vi "v5.51.vi"() -> ()   [LabVIEW 2018]
uses:
  <vilib>/DAQmx/read.llb/DAQmx Read (Analog 1D DBL NChan 1Samp).vi
  <extravilib>/ChannelInstances/Lossy Stream-c(a[.](c(dbl,dbl,dbl,dbl)),stamp,a[.](dbl),c(dbl,dbl,dbl,dbl,dbl,dbl,dbl))/Read With Abort.vi
  <extravilib>/ChannelInstances/High Speed Stream-c(a[.](c(dbl,dbl,dbl,dbl)),stamp,a[.](dbl),c(dbl,dbl,dbl,dbl,dbl,dbl,dbl))/_Read For Replicate.vi
  <extravilib>/ChannelInstances/Lossy Stream-c(a[.](c(dbl,dbl,dbl,dbl)),stamp,a[.](dbl),c(dbl,dbl,dbl,dbl,dbl,dbl,dbl))/Write With Abort.vi
  <extravilib>/ChannelInstances/Lossy Stream-c(a[.](c(dbl,dbl,dbl,dbl)),stamp,a[.](dbl),c(dbl,dbl,dbl,dbl,dbl,dbl,dbl))/EndpointRead.vi
  <extravilib>/ChannelInstances/Lossy Stream-c(a[.](c(dbl,dbl,dbl,dbl)),stamp,a[.](dbl),c(dbl,dbl,dbl,dbl,dbl,dbl,dbl))/Endpoint.vi
  <extravilib>/ChannelInstances/Lossy Stream-c(a[.](c(dbl,dbl,dbl,dbl)),stamp,a[.](dbl),c(dbl,dbl,dbl,dbl,dbl,dbl,dbl))/Instantiate.vi
  <extravilib>/ChannelInstances/Lossy Stream-c(a[.](c(dbl,dbl,dbl,dbl)),stamp,a[.](dbl),c(dbl,dbl,dbl,dbl,dbl,dbl,dbl))/)Channel.vi
  <resource>/ChannelSupport/_ChannelSupport/WaitIfNeeded.vi
  <extravilib>/ChannelInstances/High Speed Stream-c(a[.](c(dbl,dbl,dbl,dbl)),stamp,a[.](dbl),c(dbl,dbl,dbl,dbl,dbl,dbl,dbl))/Instantiate.vi
  <extravilib>/ChannelInstances/High Speed Stream-c(a[.](c(dbl,dbl,dbl,dbl)),stamp,a[.](dbl),c(dbl,dbl,dbl,dbl,dbl,dbl,dbl))/)Channel.vi
  <extravilib>/ChannelInstances/High Speed Stream-c(a[.](c(dbl,dbl,dbl,dbl)),stamp,a[.](dbl),c(dbl,dbl,dbl,dbl,dbl,dbl,dbl))/Abort Signal/Init Signal.vi
  <vilib>/Utility/file.llb/Write Delimited Spreadsheet (string).vi
  <vilib>/DAQmx/create/channels.llb/DAQmx Create Channel (AI-Temperature-Thermocouple).vi
  <vilib>/DAQmx/configure/timing.llb/DAQmx Timing (Sample Clock).vi
  <vilib>/DAQmx/miscellaneous.llb/DAQmx Fill In Error Info.vi
  <extravilib>/ChannelInstances/High Speed Stream-c(a[.](c(dbl,dbl,dbl,dbl)),stamp,a[.](dbl),c(dbl,dbl,dbl,dbl,dbl,dbl,dbl)).lvlib
  <resource>/objmgr/daqmx.rc
  <extravilib>/ChannelInstances/Lossy Stream-c(a[.](c(dbl,dbl,dbl,dbl)),stamp,a[.](dbl),c(dbl,dbl,dbl,dbl,dbl,dbl,dbl)).lvlib
panel:
  out "Thermal Power [kJ/s]":dbl
  out "Equivalence Ratio":dbl
  out "Total Air Flow Required for \nStoichiometric Combustion":dbl
  out "Mixture AFR":dbl
  out "Total Fuel Flow [g/s]":dbl
  out "Total Air Flow [g/s]":dbl
  in  "Rig Temperature Tab Box":enum32{"Rig Temps Live", "Alarm Thresholds"}(tab)
  out "Rig Temperatures":T1
  in  "Rig Alarm Thresholds":T1
  out "DAQ Current Time":timestamp format="%<%X>T"
  in  "UI Refresh Rate (Hz)":u32=1 min=1 max=500 step=1
  out "Line Pressures":T2(graph)
  in  "Boondoggle":dbl(slide) scale=0.0..10.0
  out "Line Temperatures":T2(graph)
  in  "Species List":string[][](table)=[["Custom", "9999999999", ""], ["Methanol", "6.47", "19.93"], ["Butanol", "11.2", "33.075"], ["Propane", "15.67", "46.35"], ["Methane", "13.19", "50.00"], ["Hydrogen", "34.3", "119.96"], ["Ammonia", "6.0466", "22.5"], ["Pentane", "15.32", "45.36"], ["Butane", "14.98", "45.75"], ["Hexane", "15.24", "44.75"], ["Ethanol", "9", "26.70"], ["Empty (Not Used)", "0", "0"]]
  in  "Lines Tab Control\n(Don't delete)":enum32{"Live Data", "AFR Info", "Setup Lines"}(tab)
  out "Flowrate Data":T3(array[cluster])
  out "AFR Display":T4(array[cluster])
  in  "Line Setup":T5(array[cluster])
  out "Actual Sample Rate":dbl
  out "Export Timestamp":timestamp format="%<%H:%M:%S>T"
  out "UI Timestamp":timestamp format="%<%X\n%x>T"
  in  "file path (dialog if empty)":path
  out "Export Loop Status":T6(ring)
  in  "Start Recording?":bool
  in  "Stop Recording?":bool
  out "Aquisition\nLoop Status":T7(ring)
  in  "OK Button":bool
  in  "DAQ Properties":cluster{"Sample Rate [Hz]":dbl}={"Sample Rate [Hz]"=1.0} {"Sample Rate [Hz]" min=1.0 max=500.0 step=1.0}
  # "Rig Temperatures [ °C]"
  # "Rig Alarm Thresholds [ °C]"
  # "Live \n Live Line Data"
  # "Air-to-Fuel Ratios for each Line"
  # "Line Setup"
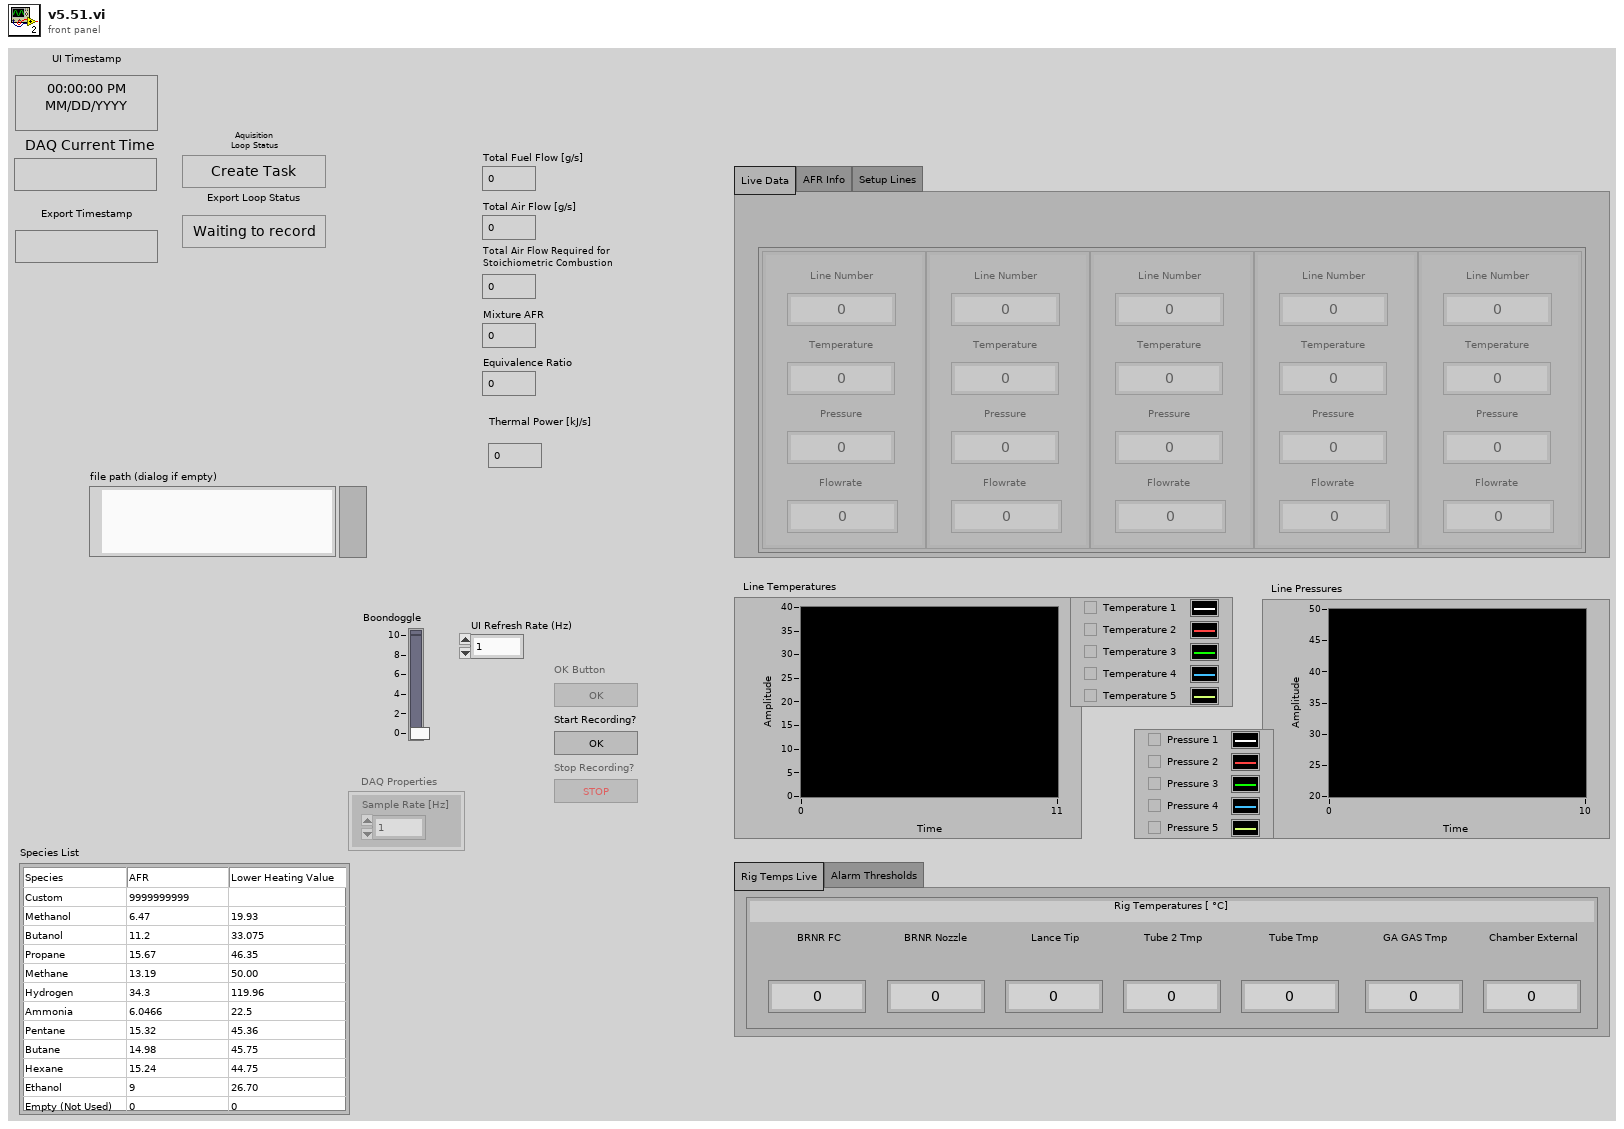
[diagram p1: front panel]
types:
  T1 = cluster{"BRNR FC":dbl, "BRNR Nozzle":dbl, "Lance Tip":dbl, "Tube 2 Tmp":dbl, "Tube Tmp":dbl, "GA GAS Tmp":dbl, "Chamber External":dbl}
  T2 = cluster{"[0]":dbl, "[1]":dbl, "[2]":dbl, "[3]":dbl, "[4]":dbl}
  T3 = cluster{"Line Number":dbl, "Temperature":dbl, "Pressure":dbl, "Flowrate":dbl}[]
  T4 = cluster{"Line Number":i32, "AFR":dbl, "Species":enum16{"Empty (Not used)", "Custom", "Air", "Methanol", "Ethanol", "Butanol", "Propane", "Methane", "Hydrogen", "Pentane", "Butane", "Hexane"}}[]
  T5 = cluster{"Custom AFR":dbl, "Species":enum16{"Empty (Not used)", "Custom", "Air", "Methanol", "Ethanol", "Butanol", "Propane", "Methane", "Hydrogen", "Pentane", "Butane", "Hexane"}, "Custom Lower Heating Value [kJ/kg]":dbl}[]
  T6 = enum16{"Waiting to record", "Creating Spreadsheet", "Recording", "Finished Recording"}
  T7 = enum16{"Create Task", "Change Settings", "Check Settings", "Read Data", "End Task"}
  T8 = enum8{"Enabled", "Disabled", "Disabled and Grayed Out"}
  T9 = cluster{"Flowrate Data":cluster{"Line Number":dbl, "Temperature":dbl, "Pressure":dbl, "Flowrate":dbl}[], "Current Time":timestamp, "DAQmx Data":dbl[], "Rig Temperatures":cluster{"BRNR FC":dbl, "BRNR Nozzle":dbl, "Lance Tip":dbl, "Tube 2 Tmp":dbl, "Tube Tmp":dbl, "GA GAS Tmp":dbl, "Chamber External Temp":dbl}}
  T10 = cluster{"BRNR FC":dbl, "BRNR Nozzle":dbl, "Lance Tip":dbl, "Tube 2 Tmp":dbl, "Tube Tmp":dbl, "GA GAS Tmp":dbl, "Chamber External Temp":dbl}
  T11 = typedef "High Speed Stream-c(a[.](c(dbl,dbl,dbl,dbl)),stamp,a[.](dbl),c(dbl,dbl,dbl,dbl,dbl,dbl,dbl)).lvlib/)Channel.ctl" = refnum<queue>
  T12 = typedef "Lossy Stream-c(a[.](c(dbl,dbl,dbl,dbl)),stamp,a[.](dbl),c(dbl,dbl,dbl,dbl,dbl,dbl,dbl)).lvlib/)Channel.ctl" = refnum<queue>
  T13 = cluster{"Line":i32, "AFR":dbl, "Species":enum16{"Empty (Not used)", "Custom", "Air", "Methanol", "Ethanol", "Butanol", "Propane", "Methane", "Hydrogen", "Pentane", "Butane", "Hexane"}}
  T14 = enum16{"Empty (Not used)", "Custom", "Air", "Methanol", "Ethanol", "Butanol", "Propane", "Methane", "Hydrogen", "Pentane", "Butane", "Hexane"}
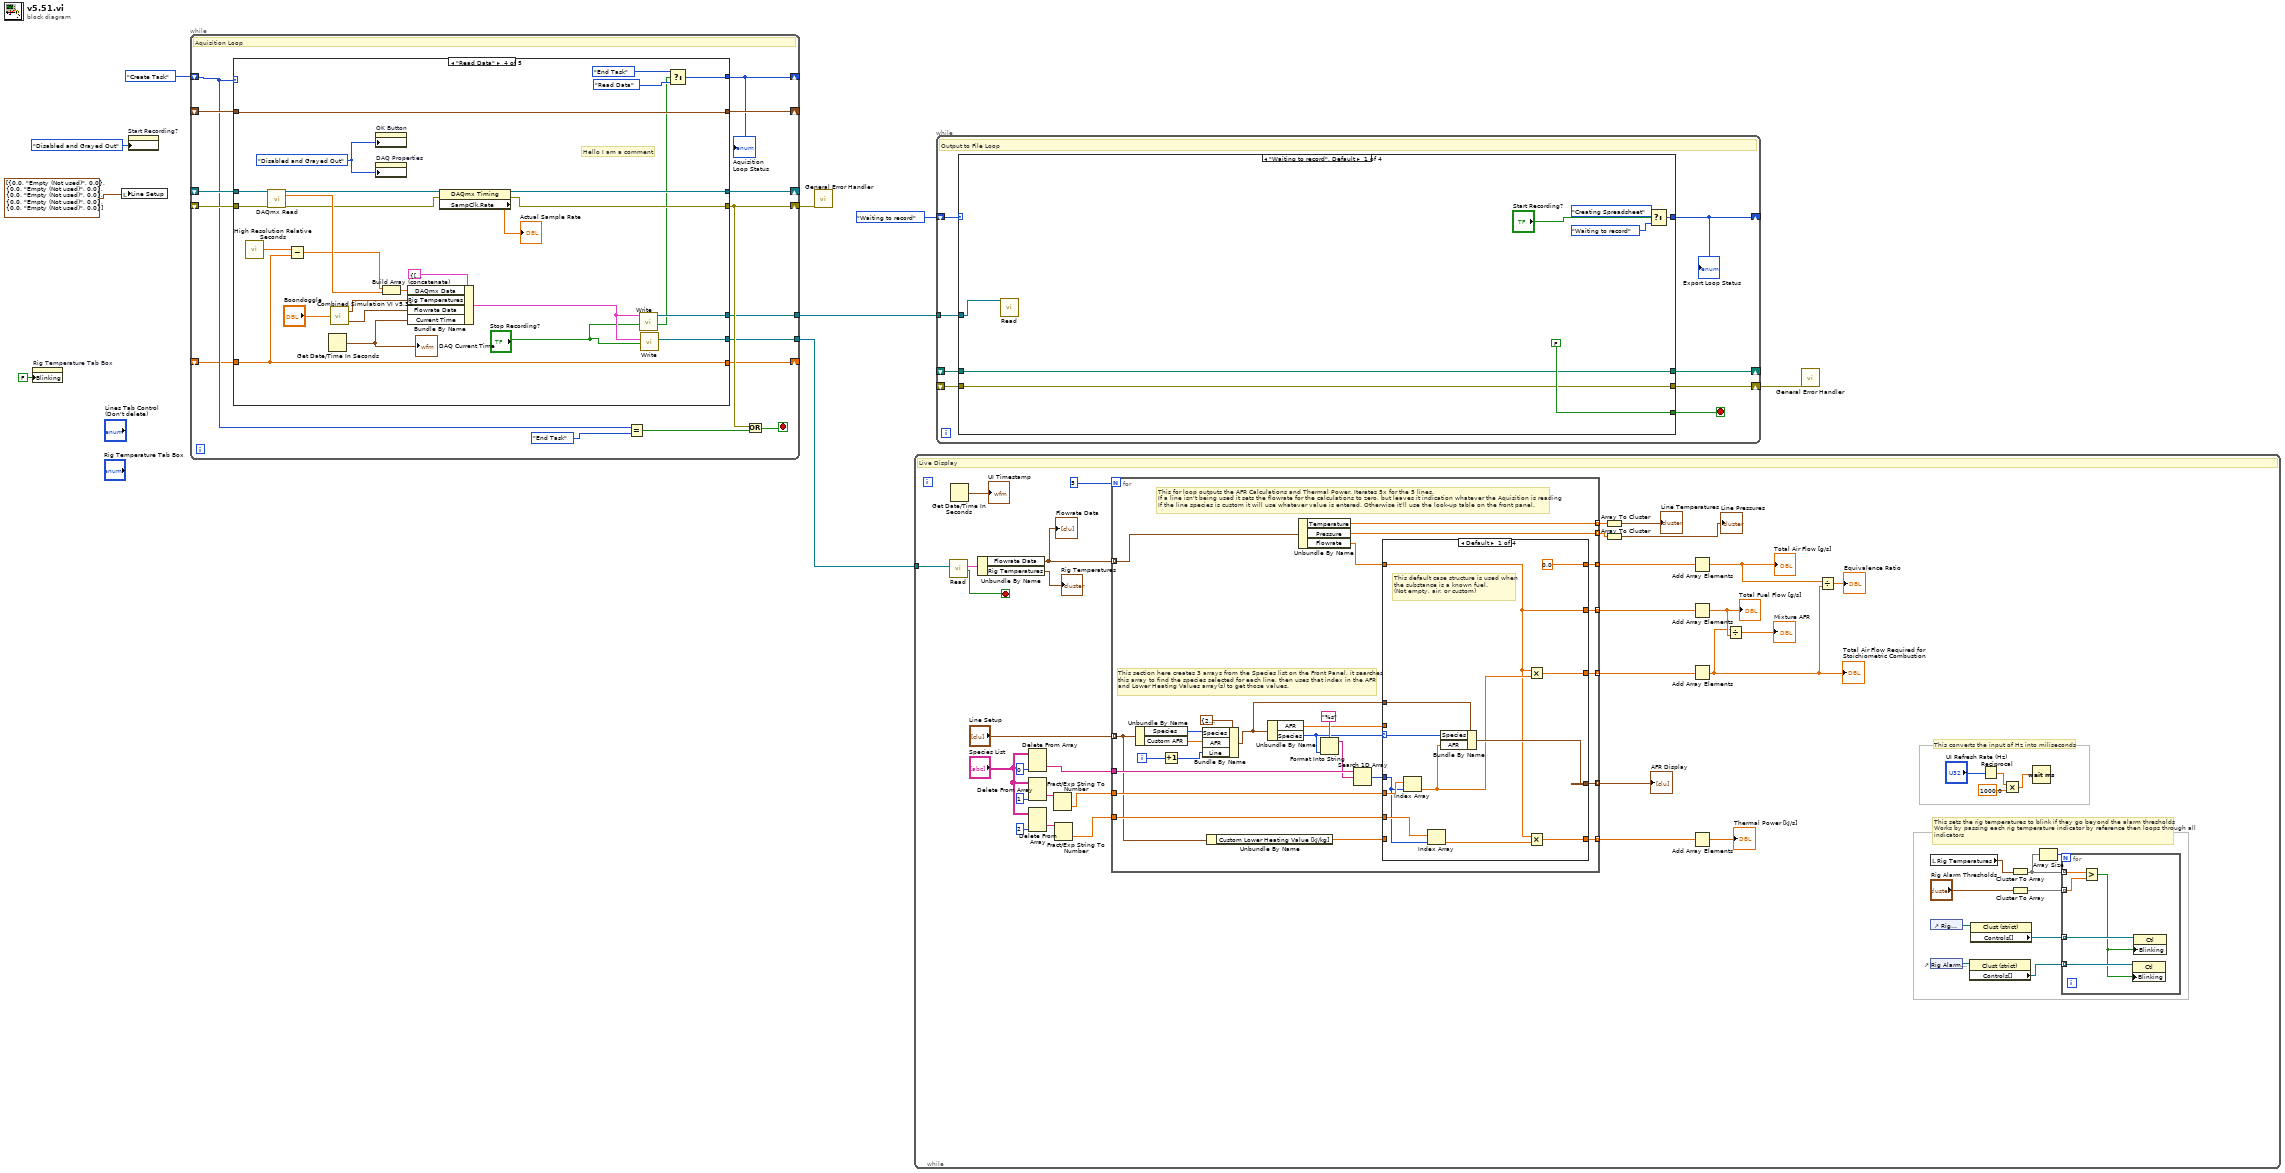
[diagram p0: block diagram]
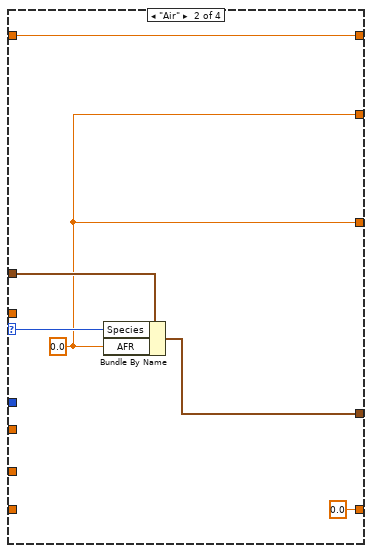
[diagram p2: hidden frame]
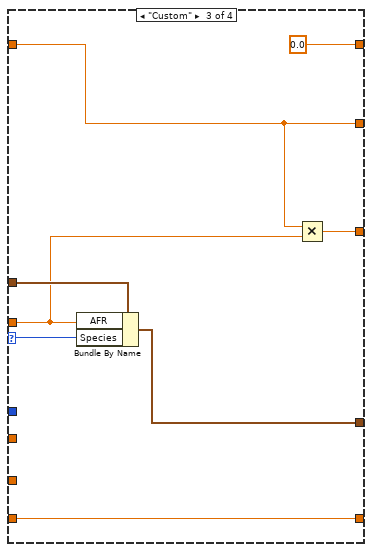
[diagram p3: hidden frame]
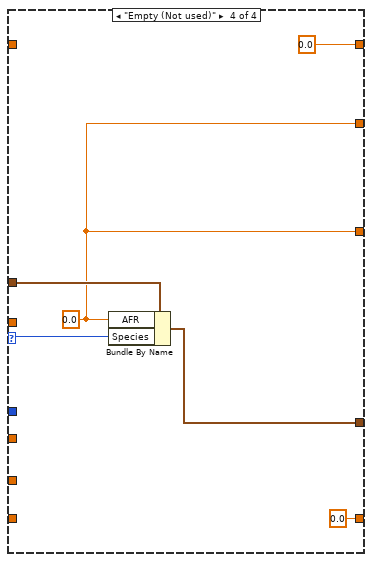
[diagram p4: hidden frame]
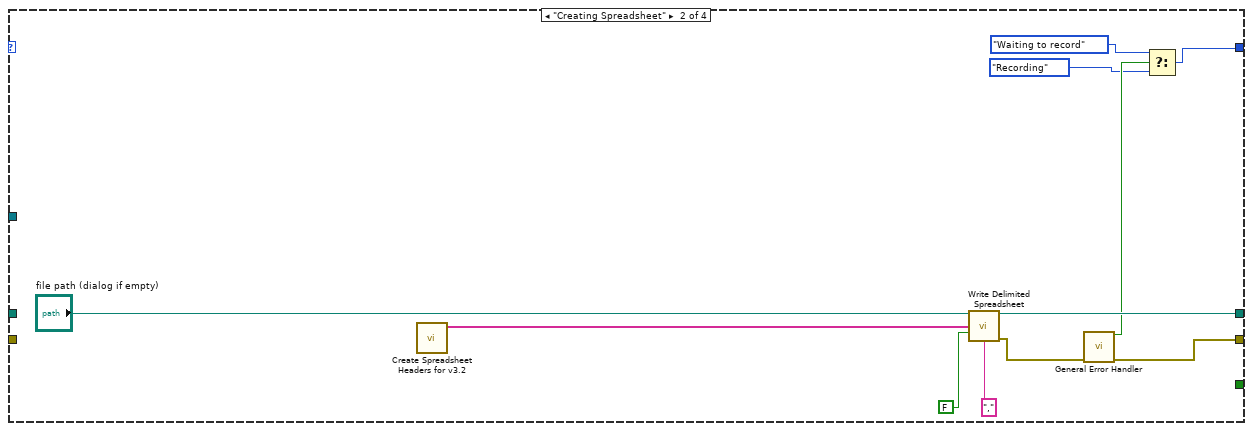
[diagram p5: hidden frame]
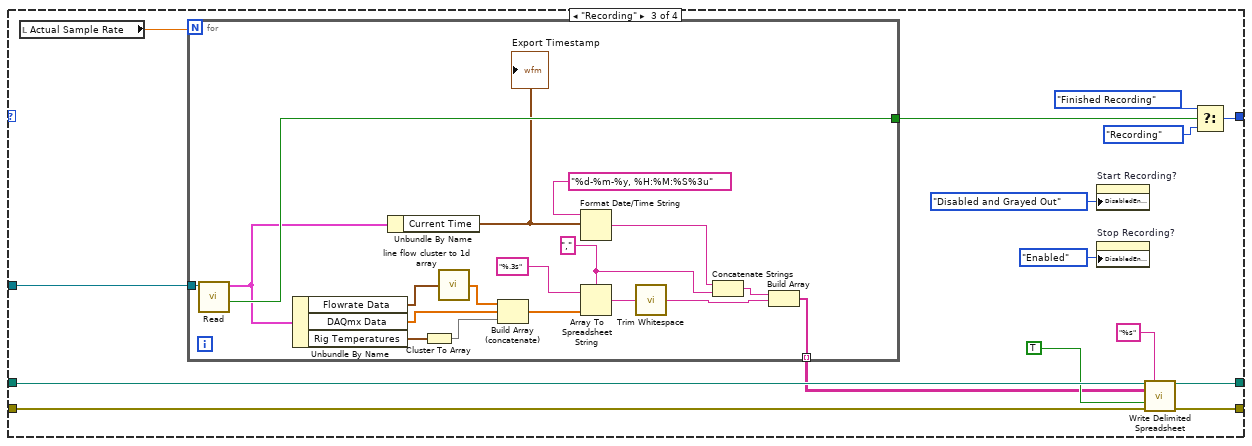
[diagram p6: hidden frame]
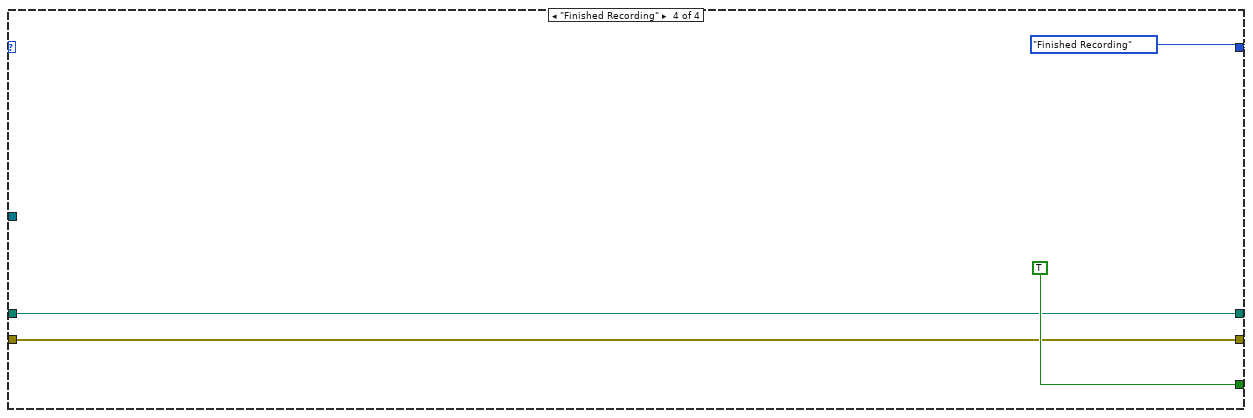
[diagram p7: hidden frame]
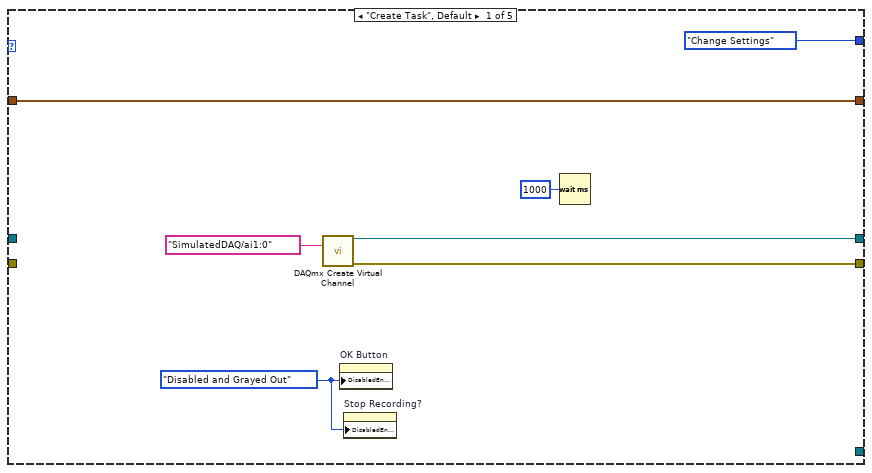
[diagram p8: hidden frame]
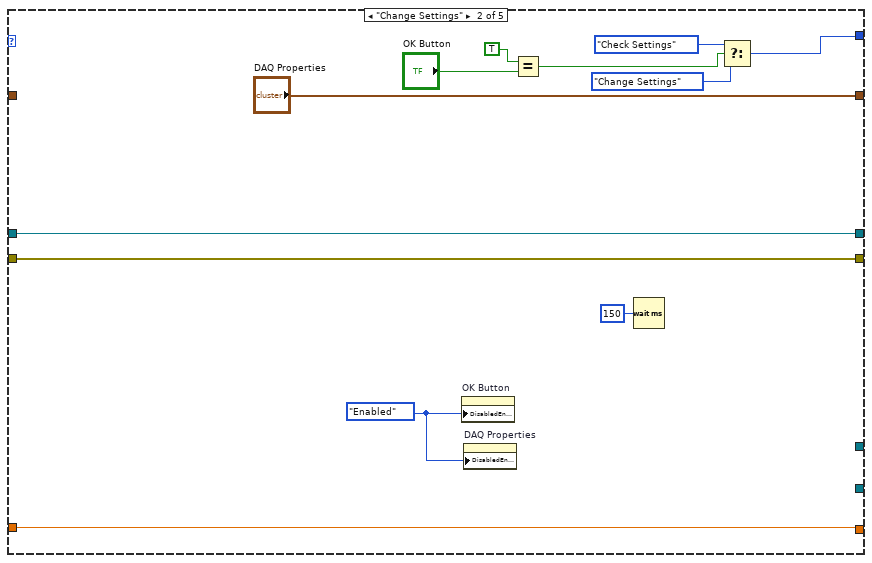
[diagram p9: hidden frame]
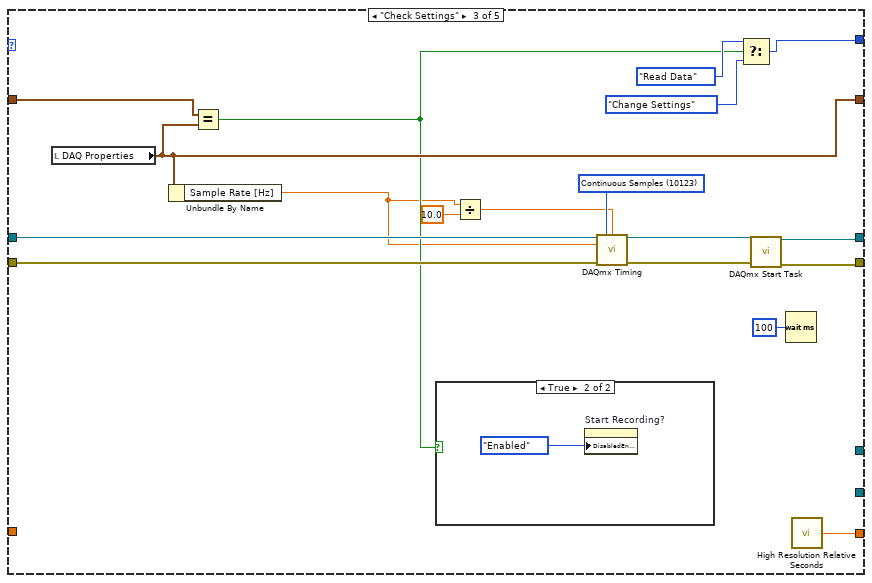
[diagram p10: hidden frame]
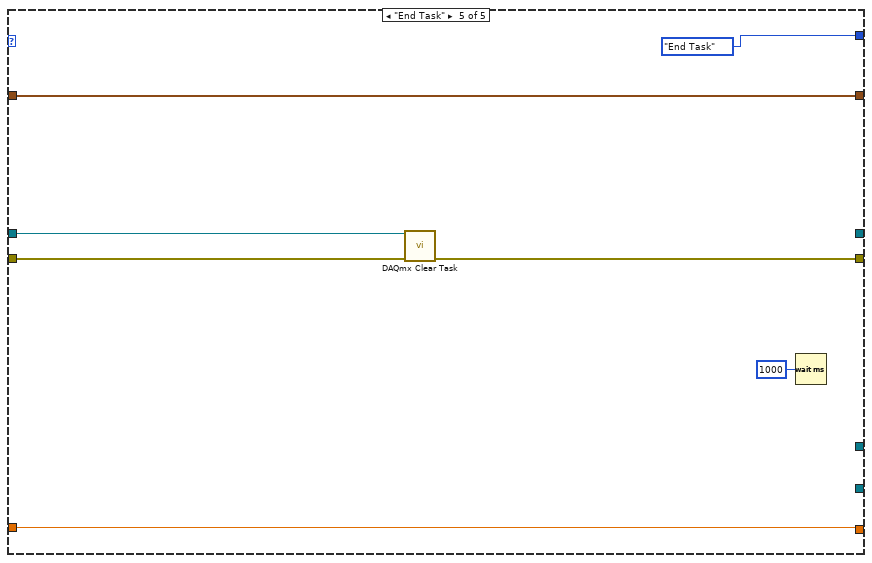
[diagram p12: hidden frame]
diagram:
  n1 = property on="Rig Temperature Tab Box" class="TabCtl (strict)"("Blinking"=FALSE) -> ()  [unwired: 2 in, 2 out]
  n2 = local write "Line Setup"(T5 [{"Custom AFR"=0.0, "Species"=enum."Empty (Not used)", "Custom Lower Heating Value [kJ/kg]"=0.0}, {"Custom AFR"=0.0, "Species"=enum."Empty (Not used)", "Custom Lower Heating Value [kJ/kg]"=0.0}, {"Custom AFR"=0.0, "Species"=enum."Empty (Not used)", "Custom Lower Heating Value [kJ/kg]"=0.0}, {"Custom AFR"=0.0, "Species"=enum."Empty (Not used)", "Custom Lower Heating Value [kJ/kg]"=0.0}, {"Custom AFR"=0.0, "Species"=enum."Empty (Not used)", "Custom Lower Heating Value [kJ/kg]"=0.0}] ("Line Setup")) -> ()
  n3 = property on="Start Recording?" class="Bool"("DisabledEnum"=T8."Disabled and Grayed Out" ("Disabled")) -> ()  [unwired: 2 in, 2 out]
  n4 = while {
    shift-right: [w19] -> _
    shift-left: T7."Create Task" -> [w15]
    shift-right: [w24] -> _
    shift-left: _ -> [w22]
    shift-right: [w18] -> w5
    shift-left: _ -> [w21]
    shift-right: [w23] -> _
    shift-left: _ -> [w20]
    tunnel: [w14] -> w7
    tunnel: [w12] -> w3
    shift-right: [w10] -> _
    shift-left: _ -> [w11]
    stop <- w13 stop-if-true
    # "Aquisition Loop"
    n5 = case shown="\"Read Data\"" w15 {
      tunnel: [w31 w43 w51 w76 _] -> w24
      tunnel: [w30 w42 w50 w77 w96] -> w18
      tunnel: [T7."Change Settings" w36 w57 w85 T7."End Task"] -> w19
      tunnel: [w27 "DAQ Properties" w54 w87 w95] -> w23
      tunnel: w22 -> [_ w43 w56 w89 w93]
      tunnel: w21 -> [_ w42 w55 w88 w92]
      tunnel: w20 -> [w27 _ w61 w87 w95]
      tunnel: [_ _ _ w81 _] -> w14
      tunnel: [_ w32 w44 w72 w90] -> w10
      tunnel: w11 -> [_ w32 _ w72 w90]
      tunnel: [_ _ _ w69 _] -> w12
      frame "Create Task", Default {
        w25 = T8."Disabled and Grayed Out" ("Disabled")
        n6 = call-poly <vilib>:"DAQmx Create Virtual Channel.vi"("physical channels"=tag "SimulatedDAQ/ai1:0") -> ("task out"=w31:refnum<k21>, "error out"=w30:errorcluster)  [unwired: 13 in]
        n7 = property on="OK Button" class="Bool"("DisabledEnum"=w25) -> ()  [unwired: 2 in, 2 out]
        n8 = property on="Stop Recording?" class="Bool"("DisabledEnum"=w25) -> ()  [unwired: 2 in, 2 out]
        n9 = Wait (ms)(milliseconds to wait=u32 1000) -> ()  [unwired: 1 out]
      }
      frame "Change Settings" {
        w33 = T8."Enabled" ("Disabled")
        n10 = property on="OK Button" class="Bool"("DisabledEnum"=w33) -> ()  [unwired: 2 in, 2 out]
        n11 = property on="DAQ Properties" class="Clust (strict)"("DisabledEnum"=w33) -> ()  [unwired: 2 in, 2 out]
        n12 = Equal?(x=TRUE, y="OK Button") -> (x = y?=w38:bool)
        n13 = Wait (ms)(milliseconds to wait=u32 150) -> ()  [unwired: 1 out]
        n14 = Select(t=T7."Check Settings", s=w38, f=T7."Change Settings") -> (s? t:f=w36:T7)
      }
      frame "Check Settings" {
        w49 = 10123 items=["Finite Samples"=10178, "Continuous Samples"=10123, "Hardware Timed Single Point"=12522] ("sample mode")
        n15 = local read "DAQ Properties"() -> (w54:cluster{"Sample Rate [Hz]":dbl})
        n16 = Unbundle By Name(w54) -> ("Sample Rate [Hz]"=w46:dbl)
        n17 = Equal?(x=w61, y=w54) -> (x = y?=w48:bool)
        n18 = case shown="True" w48 {
          frame False {
          }
          frame True {
            n19 = property on="Start Recording?" class="Bool"("DisabledEnum"=T8."Enabled" ("Disabled")) -> ()  [unwired: 2 in, 2 out]
          }
        }
        n20 = Divide(x=w46, y=10.0) -> (x/y=w45:dbl)
        n21 = call-poly <vilib>:"DAQmx Timing.vi"("task/channels in"=w56, "sample mode"=w49, "samples per channel"=w45, "rate"=w46, "error in"=w55) -> ("task out"=w53:refnum<k21>, "error out"=w52:errorcluster)  [unwired: 9 in]
        n22 = Select(t=T7."Read Data", s=w48, f=T7."Change Settings") -> (s? t:f=w57:T7)
        n23 = call <vilib>:"DAQmx Start Task.vi"("task/channels in"=w53, "error in"=w52) -> ("task out"=w51:refnum<k21>, "error out"=w50:errorcluster)  [unwired: 12 in]
        n24 = Wait (ms)(milliseconds to wait=u32 100) -> ()  [unwired: 1 out]
        n25 = call <vilib>:"High Resolution Relative Seconds.vi"() -> ("relative seconds"=w44:dbl)
      }
      frame "Read Data" {
        w80 = T8."Disabled and Grayed Out" ("Disabled")
        # "Hello I am a comment"
        n26 = call <vilib>:"High Resolution Relative Seconds.vi"() -> ("relative seconds"=w74:dbl)
        n27 = call-poly <vilib>:"DAQmx Read.vi"("task/channels in"=w89, "error in"=w88) -> ("task out"=w78:refnum<k21>, "data"=w83:dbl[], "error out"=w75:errorcluster)  [unwired: 11 in]
        n28 = Subtract(x=w74, y=w72) -> (x-y=w73:dbl)
        n29 = Get Date/Time In Seconds() -> (seconds since 1Jan1904=w64:timestamp)
        "DAQ Current Time" <- w64
        n30 = call "Combined Simulation VI v5.31.vi"("Boondoggle Input"="Boondoggle") -> ("Rig Temperatures Cluster"=w63:T10, "Line Data (Array of Clusters)"=w65:T3)
        n31 = property on="OK Button" class="Bool"("DisabledEnum"=w80) -> ()  [unwired: 2 in, 2 out]
        n32 = property on="DAQ Properties" class="Clust (strict)"("DisabledEnum"=w80) -> ()  [unwired: 2 in, 2 out]
        n33 = Build Array (concatenate)(w73, w83) -> (w67:dbl[])
        n34 = Bundle By Name(cluster=T9 {"Flowrate Data"=[{"Line Number"=1.0, "Temperature"=17.480721541683437, "Pressure"=24.0, "Flowrate"=0.0}, {"Line Number"=2.0, "Temperature"=21.850901927104296, "Pressure"=30.0, "Flowrate"=0.0}, {"Line Number"=3.0, "Temperature"=26.221082312525155, "Pressure"=36.0, "Flowrate"=0.0}, {"Line Number"=4.0, "Temperature"=30.591262697946018, "Pressure"=42.00000000000001, "Flowrate"=0.0}, {"Line Number"=5.0, "Temperature"=34.96144308336687, "Pressure"=48.0, "Flowrate"=0.0}], "Current Time"=timestamp(0 s since 1904-01-01), "DAQmx Data"=[], "Rig Temperatures"={"BRNR FC"=0.0, "BRNR Nozzle"=0.0, "Lance Tip"=0.0, "Tube 2 Tmp"=0.0, "Tube Tmp"=0.0, "GA GAS Tmp"=0.0, "Chamber External Temp"=0.0}}, "DAQmx Data"=w67, "Rig Temperatures"=w63, "Flowrate Data"=w65, "Current Time"=w64) -> (w79:T9)
        n35 = property class="DAQmx Timing"(reference=w78, error in=w75) -> (reference out=w76:refnum<k21>, error out=w77:errorcluster, "SampClk.Rate"=→"Actual Sample Rate":dbl)
        n36 = call <extravilib>:"Write.vi"("last element? (F)"="Stop Recording?", "element"=w79) -> ("done?"=w68:bool, "channel"=w81:T11)  [unwired: 7 in, 1 out]
        n37 = call <extravilib>:"Write.vi"("last element? (F)"="Stop Recording?", "element"=w79) -> ("channel"=w69:T12)  [unwired: 7 in, 2 out]
        n38 = Select(t=T7."End Task", s=w68, f=T7."Read Data") -> (s? t:f=w85:T7)
      }
      frame "End Task" {
        n39 = call <vilib>:"DAQmx Clear Task.vi"("task in"=w93, "error in"=w92) -> ("error out"=w96:errorcluster)  [unwired: 13 in]
        n40 = Wait (ms)(milliseconds to wait=u32 1000) -> ()  [unwired: 1 out]
      }
    }
    "Aquisition\nLoop Status" <- w19
    n41 = Equal?(x=w15, y=T7."End Task") -> (x = y?=w16:bool)
    n42 = Or(x=w18, y=w16) -> (x .or. y?=w13:bool)
  }
  n43 = call <vilib>:"General Error Handler.vi"("error in (no error)"=w5) -> ()  [unwired: 10 in, 5 out]
  n44 = while {
    tunnel: w3 -> [w140]
    stop <- w137 stop-if-true
    # "This converts the input of Hz into miliseconds"
    # "This sets the rig temperatures to blink if they go beyond the alarm thresholds\nWorks by passing each rig temperature indicator by reference then loops through all indicators"
    # "Live Display"
    n45 = call <extravilib>:"Read.vi"("channel"=w140) -> ("last element?"=w137:bool, "element"=w139:T9)  [unwired: 5 in, 4 out]
    n46 = Get Date/Time In Seconds() -> (seconds since 1Jan1904=→"UI Timestamp":timestamp)
    n47 = Unbundle By Name(w139) -> ("Flowrate Data"=w115:T3, "Rig Temperatures"=→"Rig Temperatures":T10)
    "Flowrate Data" <- w115
    n48 = Delete From Array(array="Species List", index (col)=0) -> (deleted portion=w128:string[])  [unwired: 2 in, 1 out]
    n49 = Delete From Array(array="Species List", index (col)=1 ("disabled index (col)")) -> (deleted portion=w129:string[])  [unwired: 2 in, 1 out]
    n50 = Delete From Array(array="Species List", index (col)=2 ("disabled index (col)")) -> (deleted portion=w100:string[])  [unwired: 2 in, 1 out]
    n51 = Fract/Exp String To Number(string=w129) -> (number=w130:dbl[])  [unwired: 3 in, 1 out]
    n52 = Fract/Exp String To Number(string=w100) -> (number=w99:dbl[])  [unwired: 3 in, 1 out]
    n53 = for {
      N: 5 -> [_]
      tunnel: w128 -> [w170]
      tunnel: w130 -> [w167]
      tunnel: "Line Setup" -> [w148] mode=indexing
      tunnel: [w158] -> w132 mode=indexing
      tunnel: w115 -> [w152] mode=indexing
      tunnel: [w157] -> w123 mode=indexing
      tunnel: [w156] -> w120 mode=indexing
      tunnel: [w154] -> w118 mode=indexing
      tunnel: [w153] -> w117 mode=indexing
      tunnel: [w151] -> w116 mode=indexing
      tunnel: w99 -> [w150]
      tunnel: [w149] -> w97 mode=indexing
      i -> [w160]
      # "This section here creates 3 arrays from the Species list on the Front Panel, it searches \nthis array to find the species selected for each line, then uses that index in the AFR \nand Lower Heating Values array(s) to get those values."
      # "This for loop outputs the AFR Calculations and Thermal Power. Iterates 5x for the 5 lines.\nIf a line isn't being used it sets the flowrate for the calculations to zero, but leaves it indication whatever the Aquisition is reading\nIf the line species is custom it will use whatever value is entered. Otherwise it'll use the look-up table on the front panel."
      n54 = Unbundle By Name(w148) -> ("Species"=w164:T14, "Custom AFR"=w163:dbl)
      n55 = Increment(x=w160) -> (x+1=w161:i32)
      n56 = Bundle By Name(cluster=T13 {"Line"=2, "AFR"=1.0, "Species"=enum."Butane"} ("AFR Inputs"), "Species"=w164, "AFR"=w163, "Line"=w161) -> (w159:T13)
      n57 = Unbundle By Name(w148) -> ("Custom Lower Heating Value [kJ/kg]"=w147:dbl)
      n58 = Unbundle By Name(w159) -> ("AFR"=w168:dbl, "Species"=w165:T14)
      n59 = Unbundle By Name(w152) -> ("Temperature"=w157:dbl, "Pressure"=w156:dbl, "Flowrate"=w155:dbl)
      n60 = Format Into String(format string="%s", w165) -> (resulting string=w169:string)  [unwired: 2 in, 1 out]
      n61 = Search 1D Array(1D array=w170, element=w169) -> (index of element=w166:i32)  [unwired: 1 in]
      n62 = case shown="Default" w165 {
        selector: w165 -> [w182 w189 w195 w201]
        tunnel: w168 -> [_ _ w193 _]
        tunnel: w167 -> [w183 _ _ _]
        tunnel: w166 -> [w175 _ _ _]
        tunnel: [w180 w188 w197 w203] -> w158
        tunnel: w159 -> [w181 w187 w196 w202]
        tunnel: w155 -> [w174 w186 w191 _]
        tunnel: [w178 w185 w192 w200] -> w154
        tunnel: [w174 w185 w191 w200] -> w153
        tunnel: [0.0 ("Flowrate") w186 0.0 ("Flowrate") 0.0 ("Flowrate")] -> w151
        tunnel: w150 -> [w176 _ _ _]
        tunnel: [w172 0.0 w190 0.0] -> w149
        tunnel: w147 -> [_ _ w190 _]
        frame Default {
          # "This default case structure is used when\nthe substance is a known fuel.\n(Not empty, air, or custom)"
          n63 = Index Array(array=w183, index=w175) -> (element=w179:dbl)
          n64 = Index Array(array=w176, index=w175) -> (element=w173:dbl)
          n65 = Bundle By Name(cluster=w181, "Species"=w182, "AFR"=w179) -> (w180:T13)
          n66 = Multiply(x=w174, y=w179) -> (x*y=w178:dbl)
          n67 = Multiply(x=w174, y=w173) -> (x*y=w172:dbl)
        }
        frame "Air" {
          w185 = 0.0 ("AFR")
          n68 = Bundle By Name(cluster=w187, "Species"=w189, "AFR"=w185) -> (w188:T13)
        }
        frame "Custom" {
          n69 = Bundle By Name(cluster=w196, "AFR"=w193, "Species"=w195) -> (w197:T13)
          n70 = Multiply(x=w191, y=w193) -> (x*y=w192:dbl)
        }
        frame "Empty (Not used)" {
          w200 = 0.0 ("AFR")
          n71 = Bundle By Name(cluster=w202, "AFR"=w200, "Species"=w201) -> (w203:T13)
        }
      }
    }
    "AFR Display" <- w132
    n72 = Array To Cluster(array=w120) -> (cluster=→"Line Pressures":T2)
    n73 = Array To Cluster(array=w123) -> (cluster=→"Line Temperatures":T2)
    n74 = Add Array Elements(numeric array=w116) -> (sum=w103:dbl)
    "Total Air Flow [g/s]" <- w103
    n75 = Add Array Elements(numeric array=w117) -> (sum=w121:dbl)
    "Total Fuel Flow [g/s]" <- w121
    n76 = Add Array Elements(numeric array=w118) -> (sum=w104:dbl)
    "Total Air Flow Required for \nStoichiometric Combustion" <- w104
    n77 = Add Array Elements(numeric array=w97) -> (sum=→"Thermal Power [kJ/s]":dbl)
    n78 = Divide(x=w104, y=w121) -> (x/y=→"Mixture AFR":dbl)
    n79 = Divide(x=w103, y=w104) -> (x/y=→"Equivalence Ratio":dbl)
    n80 = local read "Rig Temperatures"() -> (w112:T1)
    n81 = control-ref of="Rig Temperatures"() -> (w108:refnum<vi>)
    n82 = control-ref of="Rig Alarm Thresholds"() -> (w106:refnum<vi>)
    n83 = property class="Clust (strict)"(reference=w106) -> ("Controls[]"=w105:refnum<vi>[])  [unwired: 1 in, 2 out]
    n84 = property class="Clust (strict)"(reference=w108) -> ("Controls[]"=w107:refnum<vi>[])  [unwired: 1 in, 2 out]
    n85 = Reciprocal(x="UI Refresh Rate (Hz)") -> (1/x=w134:dbl)
    n86 = Multiply(x=w134, y=1000.0) -> (x*y=w133:dbl)
    n87 = Cluster To Array(cluster=w112) -> (array=w109:dbl[])
    n88 = Cluster To Array(cluster="Rig Alarm Thresholds") -> (array=w111:dbl[])
    n89 = Wait (ms)(milliseconds to wait=w133) -> ()  [unwired: 1 out]
    n90 = Array Size(array=w109) -> (size(s)=w110:i32)
    n91 = for {
      N: w110 -> [_]
      tunnel: w111 -> [w145] mode=indexing
      tunnel: w109 -> [w146] mode=indexing
      tunnel: w107 -> [w143] mode=indexing
      tunnel: w105 -> [w144] mode=indexing
      n92 = Greater?(x=w146, y=w145) -> (0:w142:bool)
      n93 = property on="Property Node" class="Ctl"(reference=w144, "Blinking"=w142) -> ()  [unwired: 1 in, 2 out]
      n94 = property on="Property Node" class="Ctl"(reference=w143, "Blinking"=w142) -> ()  [unwired: 1 in, 2 out]
    }
  }
  n95 = while {
    shift-right: [w211] -> _
    shift-left: T6."Waiting to record" -> [w210]
    tunnel: w7 -> [w208]
    shift-right: [w206] -> _
    shift-left: _ -> [w207]
    shift-right: [w205] -> w6
    shift-left: _ -> [w204]
    stop <- w209 stop-if-true
    # "Output to File Loop"
    n96 = case shown="\"Waiting to record\", Default" w210 {
      tunnel: [w216 w222 w244 T6."Finished Recording"] -> w211
      tunnel: [FALSE _ _ TRUE] -> w209
      tunnel: w208 -> [w212 _ w241 _]
      tunnel: w207 -> [w214 _ w238 w265]
      tunnel: [w214 w230 w239 w265] -> w206
      tunnel: [w213 w224 w234 w264] -> w205
      tunnel: w204 -> [w213 _ w237 w264]
      frame "Waiting to record", Default {
        n97 = call <extravilib>:"Read.vi"("channel"=w212) -> ()  [unwired: 6 in, 5 out]
        n98 = Select(t=T6."Creating Spreadsheet", s="Start Recording?", f=T6."Waiting to record") -> (s? t:f=w216:T6)
      }
      frame "Creating Spreadsheet" {
        n99 = call "Create Spreadsheet Headers for v3.2.vi"() -> ("Array"=w229:string[])  [unwired: 11 in]
        n100 = call-poly <vilib>:"Write Delimited Spreadsheet.vi"("file path (dialog if empty)"="file path (dialog if empty)", "1D data"=w229, "append to file? (new file:F)"=FALSE, "delimiter (\\t)"="," ("delimiter (\\t)")) -> ("new file path (Not A Path if cancelled)"=w230:path, "error out"=w225:errorcluster)  [unwired: 10 in]
        n101 = call <vilib>:"General Error Handler.vi"("error in (no error)"=w225) -> ("error?"=w223:bool, "error out"=w224:errorcluster)  [unwired: 10 in, 3 out]
        n102 = Select(t=T6."Waiting to record", s=w223, f=T6."Recording") -> (s? t:f=w222:T6)
      }
      frame "Recording" {
        n103 = local read "Actual Sample Rate"() -> (w231:dbl)
        n104 = for {
          N: w231 -> [_]
          tunnel: w241 -> [w262]
          tunnel: [w261] -> w240
          tunnel: [w246] -> w232 mode=indexing
          w251 = "," ("delimiter (Tab)")
          n105 = call <extravilib>:"Read.vi"("channel"=w262) -> ("done?"=w261:bool, "element"=w259:T9)  [unwired: 6 in, 3 out]
          n106 = Unbundle By Name(w259) -> ("Flowrate Data"=w260:T3, "DAQmx Data"=w257:dbl[], "Rig Temperatures"=w263:T10)
          n107 = Unbundle By Name(w259) -> ("Current Time"=w252:timestamp)
          "Export Timestamp" <- w252
          n108 = Cluster To Array(cluster=w263) -> (array=w258:dbl[])
          n109 = call "line flow cluster to 1d array.vi"("Flowrate Data"=w260) -> ("Array"=w256:dbl[])
          n110 = Build Array (concatenate)(w256, w257, w258) -> (w249:dbl[])
          n111 = Format Date/Time String(time format string (%c)="%d-%m-%y, %H:%M:%S%3u", seconds (now)=w252) -> (date/time string=w250:string)  [unwired: 1 in]
          n112 = Array To Spreadsheet String(delimiter (Tab)=w251, array=w249, 3:"%.3s" ("format string")) -> (spreadsheet string=w255:string)
          n113 = call <vilib>:"Trim Whitespace.vi"("string"=w255) -> ("trimmed string"=w247:string)  [unwired: 1 in]
          n114 = Concatenate Strings(w250, w251) -> (w248:string)
          n115 = Build Array(w248, w247) -> (w246:string[])
        }
        n116 = property on="Start Recording?" class="Bool"("DisabledEnum"=T8."Disabled and Grayed Out" ("Disabled")) -> ()  [unwired: 2 in, 2 out]
        n117 = property on="Stop Recording?" class="Bool"("DisabledEnum"=T8."Enabled" ("Disabled")) -> ()  [unwired: 2 in, 2 out]
        n118 = call-poly <vilib>:"Write Delimited Spreadsheet.vi"("file path (dialog if empty)"=w238, "format (%s)"="%s", "2D data"=w232, "append to file? (new file:F)"=TRUE, "error in (no error)"=w237) -> ("new file path (Not A Path if cancelled)"=w239:path, "error out"=w234:errorcluster)  [unwired: 9 in]
        n119 = Select(t=T6."Finished Recording", s=w240, f=T6."Recording") -> (s? t:f=w244:T6)
      }
      frame "Finished Recording" {
      }
    }
    "Export Loop Status" <- w211
  }
  n120 = call <vilib>:"General Error Handler.vi"("error in (no error)"=w6) -> ()  [unwired: 10 in, 5 out]
